vi "Get Available Sensor Sim Components.vi"(8 "error in (no error)":errorcluster, 10 "Register Info":T6) -> (0 "error out":errorcluster, 2 "Sensor Sim Components":T1, 3 "Bitfile Signature":string)   [LabVIEW 2011, in "Sensor Simulation Custom Device.lvlib"]
uses:
  Sensor Simulation Custom Device.lvlib
  <userlib>/_FPGA Interface Advanced Tools/FPGA Bitfile Utility/TypeDefs/Scalar Register Set.ctl
  <userlib>/_FPGA Interface Advanced Tools/FPGA Bitfile Utility/TypeDefs/Scalar Register.ctl
  TypeDefs/SensorSimComps.ctl
  TypeDefs/xVDT.ctl
  TypeDefs/Resolver.ctl
  <userlib>/_FPGA Interface Advanced Tools/FPGA Bitfile Utility/FPGA Bitfile Utility.lvlib
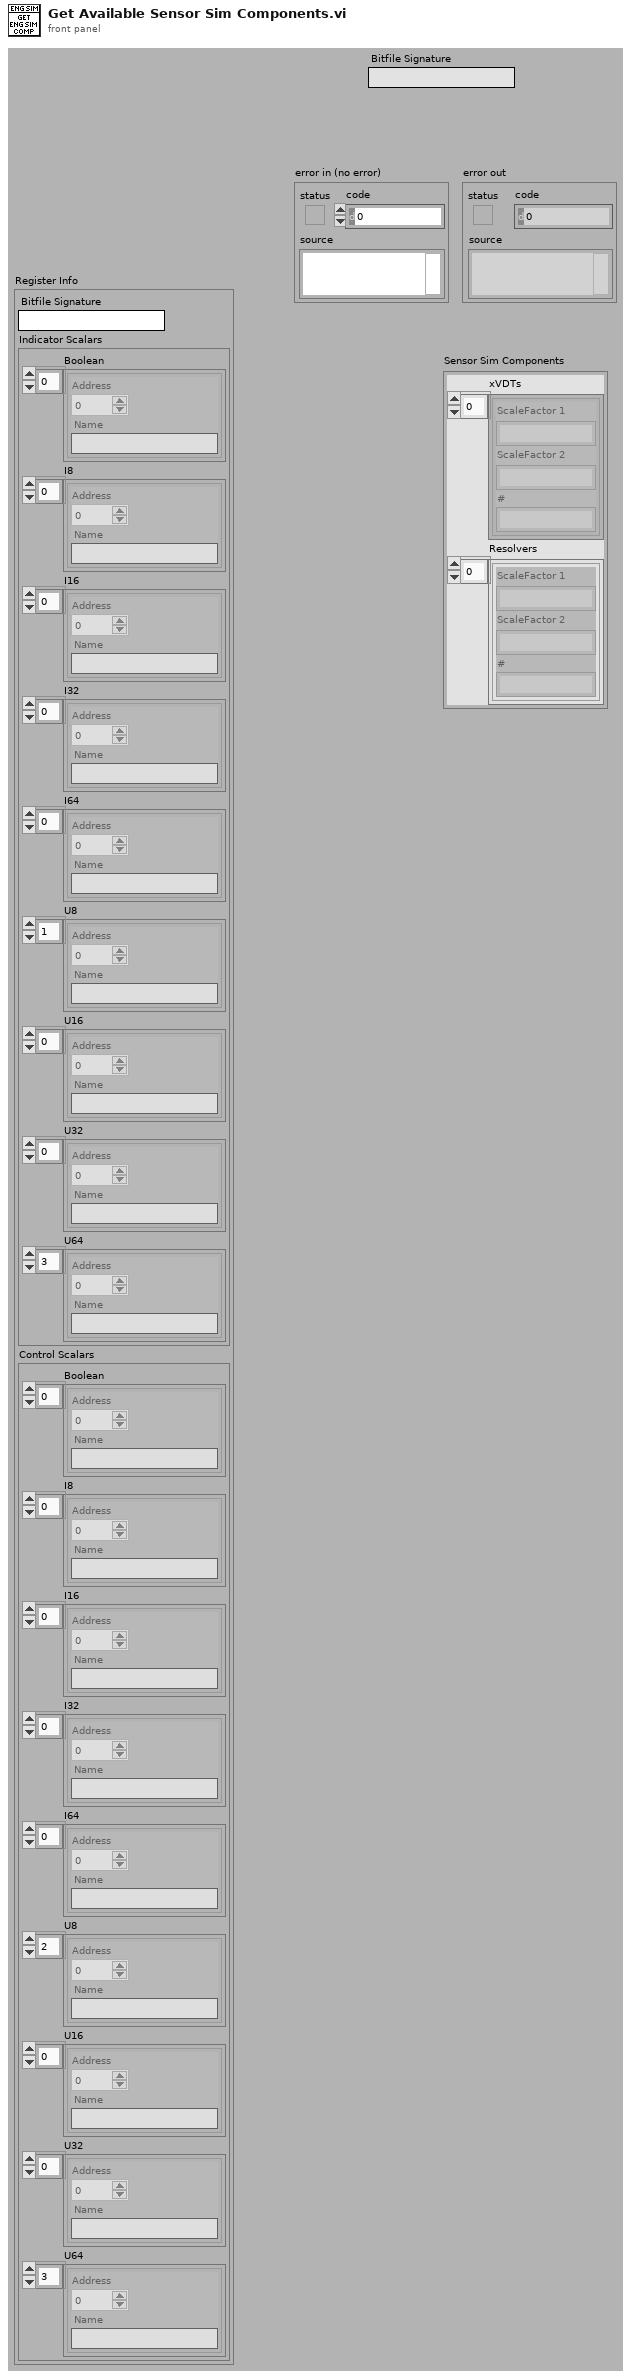
[diagram p1: front panel]
types:
  T1 = typedef "Sensor Simulation Custom Device.lvlib/SensorSimComps.ctl" = cluster{"xVDTs":T2[], "Resolvers":T3[]}
  T2 = typedef "Sensor Simulation Custom Device.lvlib/xVDT.ctl" = cluster{"ScaleFactor 1":string, "ScaleFactor 2":string, "#":string}
  T3 = typedef "Sensor Simulation Custom Device.lvlib/Resolver.ctl" = cluster{"ScaleFactor 1":string, "ScaleFactor 2":string, "#":string}
  T4 = typedef "FPGA Bitfile Utility.lvlib/Scalar Register Set.ctl" = cluster{"Boolean":T5[], "I8":T5[], "I16":T5[], "I32":T5[], "I64":T5[], "U8":T5[], "U16":T5[], "U32":T5[], "U64":T5[]}
  T5 = typedef "FPGA Bitfile Utility.lvlib/Scalar Register.ctl" = cluster{"Address":u32, "Name":string}
  T6 = cluster{"Bitfile Signature":string, "Indicator Scalars":T4, "Control Scalars":T4}
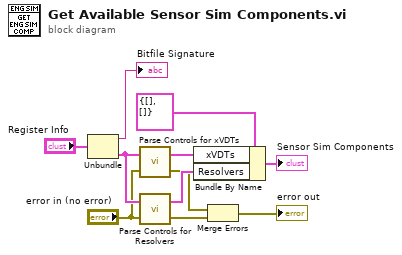
[diagram p0: block diagram]
diagram:
  n1 = Unbundle("Register Info") -> ("Bitfile Signature"=→"Bitfile Signature":string, "Control Scalars"=w6:T4)  [unwired: 1 out]
  n2 = call "Parse Controls for xVDTs.vi"("error in (no error)"="error in (no error)", "Control Scalars"=w6) -> ("error out"=w3:errorcluster, "xVDTs"=w8:T2[])
  n3 = call "Parse Controls for Resolvers.vi"("error in (no error)"="error in (no error)", "Control Scalars"=w6) -> ("error out"=w2:errorcluster, "Resolvers"=w5:T2[])
  n4 = Bundle By Name(cluster=T1 {"xVDTs"=[], "Resolvers"=[]} ("Engine Sim Components"), "xVDTs"=w8, "Resolvers"=w5) -> (→"Sensor Sim Components":T1)
  n5 = Merge Errors(w3, w2) -> (→"error out":errorcluster)
